vi "通信状态入队列.vi"(8 "错误输入（无错误）":errorcluster, 10 "发送报文":string, 11 "枚举":enum16{"打开连接", "发送数据", "读取数据", "数据处理", "关闭连接"}(ring)) -> (0 "错误输出":errorcluster)   [LabVIEW 2016, in "数据传输系统.lvlib"]
panel:
  out "data":T1
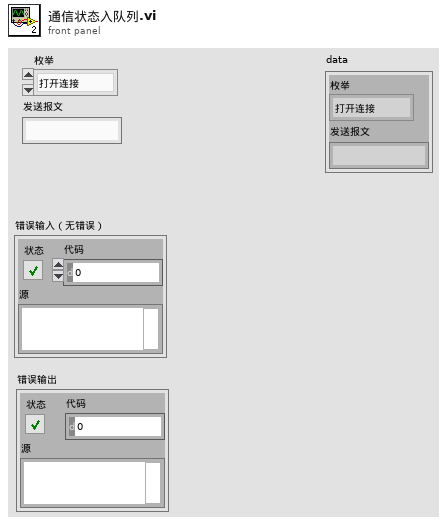
[diagram p1: front panel]
types:
  T1 = cluster{"枚举":enum16{"打开连接", "发送数据", "读取数据", "数据处理", "关闭连接"}, "发送报文":string}
  T2 = cluster{"setini":string, "sysini":string, "hechaini":string, "actualwrite":string, "actualread":string, "datasent":string, "反控命令信息队列":string, "反控与仪器交互":string}
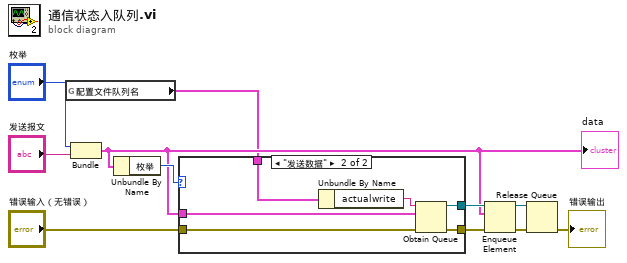
[diagram p0: block diagram]
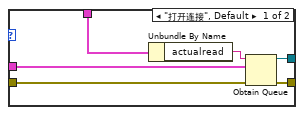
[diagram p2: hidden frame]
diagram:
  n1 = global read "全局1.vi" "配置文件队列名"() -> (w1:T2)
  n2 = Bundle("枚举"="枚举", "发送报文"="发送报文") -> (w2:T1)  [unwired: 1 in]
  "data" <- w2
  n3 = Unbundle By Name(w2) -> ("枚举"=w5:enum16{"打开连接", "发送数据", "读取数据", "数据处理", "关闭连接"})
  n4 = case shown="\"发送数据\"" w5 {
    tunnel: [w17 w23] -> w10
    tunnel: [w16 w22] -> w9
    tunnel: "错误输入（无错误）" -> [w15 w21]
    tunnel: w2 -> [w13 w19]
    tunnel: w1 -> [w12 w18]
    frame "打开连接", Default {
      n5 = Unbundle By Name(w12) -> ("actualread"=w14:string)
      n6 = Obtain Queue(name (unnamed)=w14, element data type=w13, error in (no error)=w15) -> (queue out=w17:refnum<queue>, error out=w16:errorcluster)  [unwired: 2 in, 1 out]
    }
    frame "发送数据" {
      n7 = Unbundle By Name(w18) -> ("actualwrite"=w20:string)
      n8 = Obtain Queue(name (unnamed)=w20, element data type=w19, error in (no error)=w21) -> (queue out=w23:refnum<queue>, error out=w22:errorcluster)  [unwired: 2 in, 1 out]
    }
  }
  n9 = Enqueue Element(queue=w10, element=w2, error in (no error)=w9) -> (queue out=w11:refnum<queue>, error out=w8:errorcluster)  [unwired: 1 in, 1 out]
  n10 = Release Queue(queue=w11, error in (no error)=w8) -> (error out=→"错误输出":errorcluster)  [unwired: 1 in, 2 out]
